vi "Create Physics Frame.vi"(8 "error in (no error)":errorcluster, 10 "Name":string="Physics", 11 "ODESimulator_LinearConveyor in":refnum<class "ODESimulator_LinearConveyor.lvclass">) -> (0 "error out":errorcluster, 2 "Physics Frame out":refnum<vi>, 3 "ODESimulator_LinearConveyor out":refnum<class "ODESimulator_LinearConveyor.lvclass">)   [LabVIEW 2017, in "NI_Robotics_Simulator.lvlib" / "ODESimulator_LinearConveyor.lvclass"]
uses:
  <vilib>/robotics/Simulator/Robot Factory/Conveyor/Linear/ODESimulator_LinearConveyor.lvclass
  <vilib>/robotics/Simulator/Robot Factory/Conveyor/Linear/ODESimulator_LinearConveyor.lvclass/ODESimulator_LinearConveyor.ctl
  <vilib>/robotics/Simulator/Robot Factory/Conveyor/Base/ODESimulator_Base_Conveyor.lvclass
  <vilib>/picture/3D Picture Control/NI_3D Picture Control.lvlib
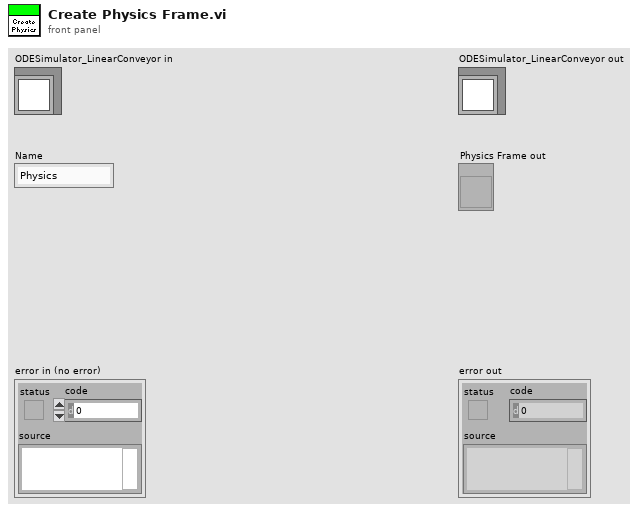
[diagram p1: front panel]
types:
  T1 = cluster{"Red":sgl, "Green":sgl, "Blue":sgl, "Alpha":sgl}
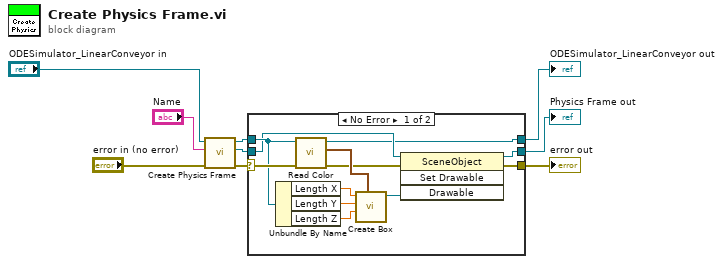
[diagram p0: block diagram]
diagram:
  n1 = call-parent "Create Physics Frame.vi"("error in (no error)"="error in (no error)", "Name"="Name", "3D_Physics_Base in"="ODESimulator_LinearConveyor in") -> ("error out"=w4:errorcluster, "Physics Frame out"=w6:refnum<vi>, "3D_Physics_Base out"=w5:refnum<class "ODESimulator_LinearConveyor.lvclass">)  [unwired: 6 in]
  n2 = case shown="No Error" w4 {
    selector: w4 -> [w16 w23]
    tunnel: w5 -> [w13 w24]
    tunnel: [w10 w24] -> w2
    tunnel: [w15 w22] -> w3
    tunnel: [w14 w23] -> w1
    tunnel: w6 -> [w12 w22]
    frame No Error {
      n3 = Unbundle By Name(w13) -> ("Length X"=w20:sgl, "Length Y"=w19:sgl, "Length Z"=w18:sgl)
      n4 = call-dynamic "Read Color.vi"("error in (no error)"=w16, "Base in"=w13) -> ("error out"=w11:errorcluster, "Color"=w21:T1, "Base out"=w10:refnum<class "ODESimulator_LinearConveyor.lvclass">)  [unwired: 7 in]
      n5 = call <vilib>:"Create Box.vi"("Color"=w21, "Length Z"=w18, "Length Y"=w19, "Length X"=w20) -> ("New Box Refnum"=w17:refnum<vi>)  [unwired: 6 in, 1 out]
      n6 = invoke class="SceneObject" method="Set Drawable"(reference=w12, error in=w11, "Drawable"=w17) -> (reference out=w15:refnum<vi>, error out=w14:errorcluster)  [unwired: 1 in, 2 out]
    }
    frame Error {
    }
  }
  "error out" <- w1
  "ODESimulator_LinearConveyor out" <- w2
  "Physics Frame out" <- w3
